vi "Read Controller Stable Response.vi"(8 "error in (no error)":errorcluster, 10 "node address (same)":u8, 11 "ProPar in":refnum<class "PL Bronkhorst ProPar.lvclass">) -> (0 "error out":errorcluster, 2 "stable response":u8, 3 "ProPar out":refnum<class "PL Bronkhorst ProPar.lvclass">)   [LabVIEW 2015, in "PL Bronkhorst ProPar.lvclass"]
doc: "Reads controller response when controller is stable (within 2% of the setpoint) of the specified <b>node</b>. Value 128 means no correction."
uses:
  PL Bronkhorst ProPar.lvclass
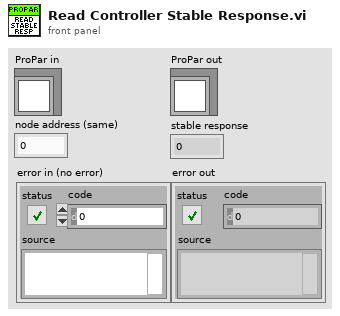
[diagram p1: front panel]
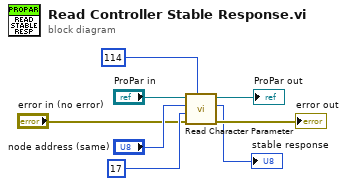
[diagram p0: block diagram]
diagram:
  n1 = call "Read Character Parameter.vi"("process number"=u8 114, "error in (no error)"="error in (no error)", "parameter number"=u8 17 ("process number"), "node"="node address (same)", "ProPar in"="ProPar in") -> ("error out"=→"error out":errorcluster, "value"=→"stable response":u8, "ProPar out"=→"ProPar out":refnum<class "PL Bronkhorst ProPar.lvclass">)  [unwired: 4 in]
